vi "HCC Build EXE Name.vi"(8 "Error In":errorcluster, 11 "Network Variable Location":i32) -> (0 "Error Out":errorcluster, 3 "Exe Name":string)   [LabVIEW 2018]
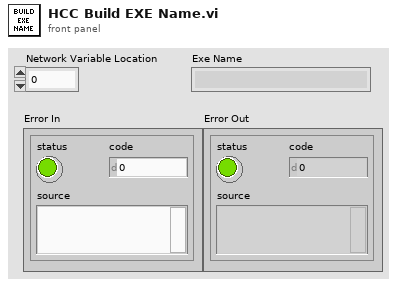
[diagram p1: front panel]
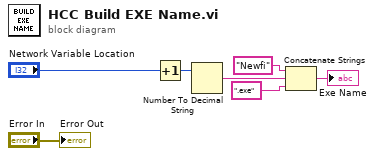
[diagram p0: block diagram]
diagram:
  n1 = Increment(x="Network Variable Location") -> (x+1=w7:i32)
  n2 = Number To Decimal String(number=w7) -> (decimal integer string=w3:string)  [unwired: 1 in]
  n3 = Concatenate Strings("Newfi" ("name or relative path"), w3, ".exe" ("string")) -> (→"Exe Name":string)
  "Error Out" <- "Error In"
